vi "setDAQ.vi"(8 "error in (no error)":errorcluster, 10 "setDAQ":variant, 11 "Instrument.LockinAPI in":refnum<class "Instrument.LockinAPI.lvclass">) -> (0 "error out":errorcluster, 3 "Instrument.LockinAPI out":refnum<class "Instrument.LockinAPI.lvclass">)   [LabVIEW 2019, in "Instrument.LockinAPI.lvclass"]
doc: "API to configure AO.\n\nIf address=\"\", this API reads from localhost\nIf address is remote lockin, you need to add this computer to allowed whitelist on the lockin computer you are trying to access."
uses:
  Instrument.LockinAPI.lvclass
  C:/Users/patrick/Documents/GitHub/Instrument-Framework/lvsrc/Instrument/Instrument.lvclass
  Typedefs/API/LockinAPI.Commands--Enum.ctl
  e567dc32-cf46-45f2-a808-c6ffdf28405d.vi
  e567dc32-cf46-45f2-a808-c6ffdf28405d.vi/d8411337-0113-42b1-a778-0f6f3735e37f.vi
  e567dc32-cf46-45f2-a808-c6ffdf28405d.vi/d8411337-0113-42b1-a778-0f6f3735e37f.vi/c320d548-fcfc-40cf-9ca8-d3a0d35e952b.vi
  e567dc32-cf46-45f2-a808-c6ffdf28405d.vi/d8411337-0113-42b1-a778-0f6f3735e37f.vi/c320d548-fcfc-40cf-9ca8-d3a0d35e952b.vi/d941d4a9-f860-4c62-9179-c22c05e25468.vi
  e567dc32-cf46-45f2-a808-c6ffdf28405d.vi/d8411337-0113-42b1-a778-0f6f3735e37f.vi/c320d548-fcfc-40cf-9ca8-d3a0d35e952b.vi/0168d3d2-3a69-4eac-93bb-a006729afd04.vi
  Instrument/Protected/Validate API method.vi
  Instrument/Private/Get RC Connection Status.vi
  Instrument/API/Send and Receive.vi
  <vilib>/Utility/Data Type/Get Type Information.vi
  <vilib>/JDP Science/JSONtext/JSON text to Variant.vi
  <vilib>/JDP Science/JSONtext/LVClass Serializer/JSONtext LVClass Serializer.lvclass
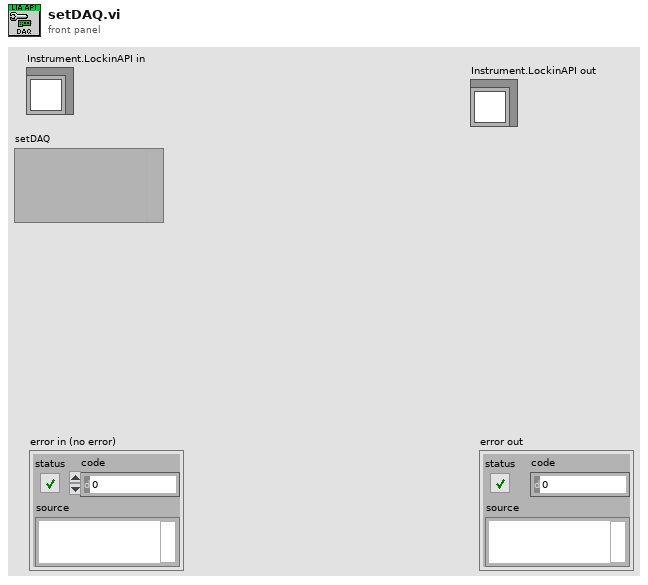
[diagram p1: front panel]
types:
  T1 = typedef "Instrument.LockinAPI.lvclass/LockinAPI.Commands--Enum.ctl" = enum16{"setAI", "setAO", "setAO_Amplitude", "setAO_DC", "setAO_Frequency", "setAO_Phase", "setAO_Function", "setAO_I+", "setREF", "setREF_Frequency", "setREF_Phase", "setREF_TC", "setREF_Roll-Off", "setDAQ", "setSampling", "setOffset", "setState", "getState", "getAO", "getAI", "getResults", "getSampling", "getAOconfig", "getREFconfig", "setInputGain", "setOutputGain", "getInputGain", "getOutputGain", "setSamplingMode", "getSamplingMode", "setSweep", "setSweepTime", "setSweepTable", "getStatus", "getSweepResults", "getSweepWaveforms", "startSweep", "stopSweep", "setAUX", "getAUX"}
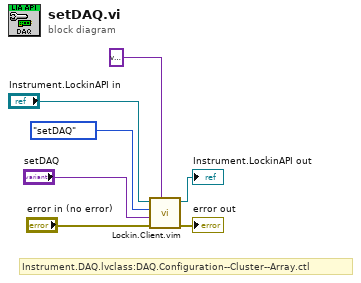
[diagram p0: block diagram]
diagram:
  # "Instrument.DAQ.lvclass:DAQ.Configuration--Cluster--Array.ctl"
  n1 = call "Lockin.Client.vim"("Data Out type"=variant, "error in (no error)"="error in (no error)", "Data"="setDAQ", "Command"=LockinAPI.Commands--Enum."setDAQ", "Instrument.LockinAPI in"="Instrument.LockinAPI in") -> ("error out"=→"error out":errorcluster, "Instrument.LockinAPI out"=→"Instrument.LockinAPI out":refnum<class "Instrument.LockinAPI.lvclass">)  [unwired: 4 in, 1 out]
